vi "Create Legend.vi"(7 "Selection":i32, 9 "Colors[] (Use Default)":u32[](array[colorbox]), 10 "Font":T1, 11 "Labels[]":string[](array[string])) -> (2 "Legend Box Size":cluster{"Width":u32, "Height":u32}, 3 "Legend out":picture)   [LabVIEW 2018, in "PieChart.lvclass"]
uses:
  PieChart.lvclass
  <vilib>/picture/picture.llb/Draw True-Color Pixmap.vi
  <vilib>/Utility/miscctls.llb/LVFontTypeDef.ctl
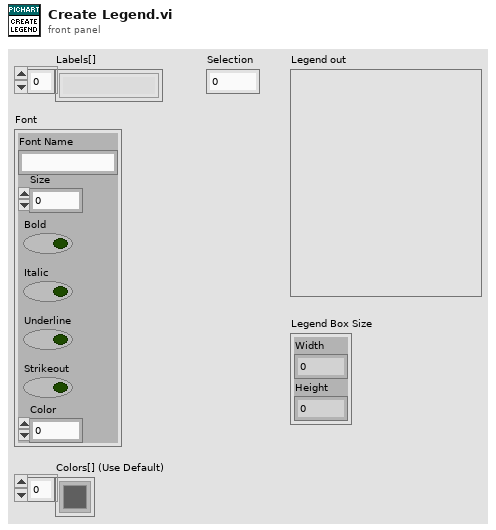
[diagram p1: front panel]
types:
  T1 = typedef "LVFontTypeDef.ctl" = cluster{"Font Name":string, "Size":u16, "Bold":bool, "Italic":bool, "Underline":bool, "Strikeout":bool, "Color":u32}
  T2 = cluster{"left":i16, "top":i16, "right":i16, "bottom":i16}
  T3 = enum16{"User-specified Font", "Application Font", "System Font", "Dialog Font"}
  T4 = cluster{"Font Name:":string, "Size":i16, "Strikeout?":bool, "Italic?":bool, "Underline?":bool, "Outline?":bool, "Shadow?":bool, "Bold?":bool}
  T5 = cluster{"left":u32, "top":u32, "right":u32, "bottom":u32}
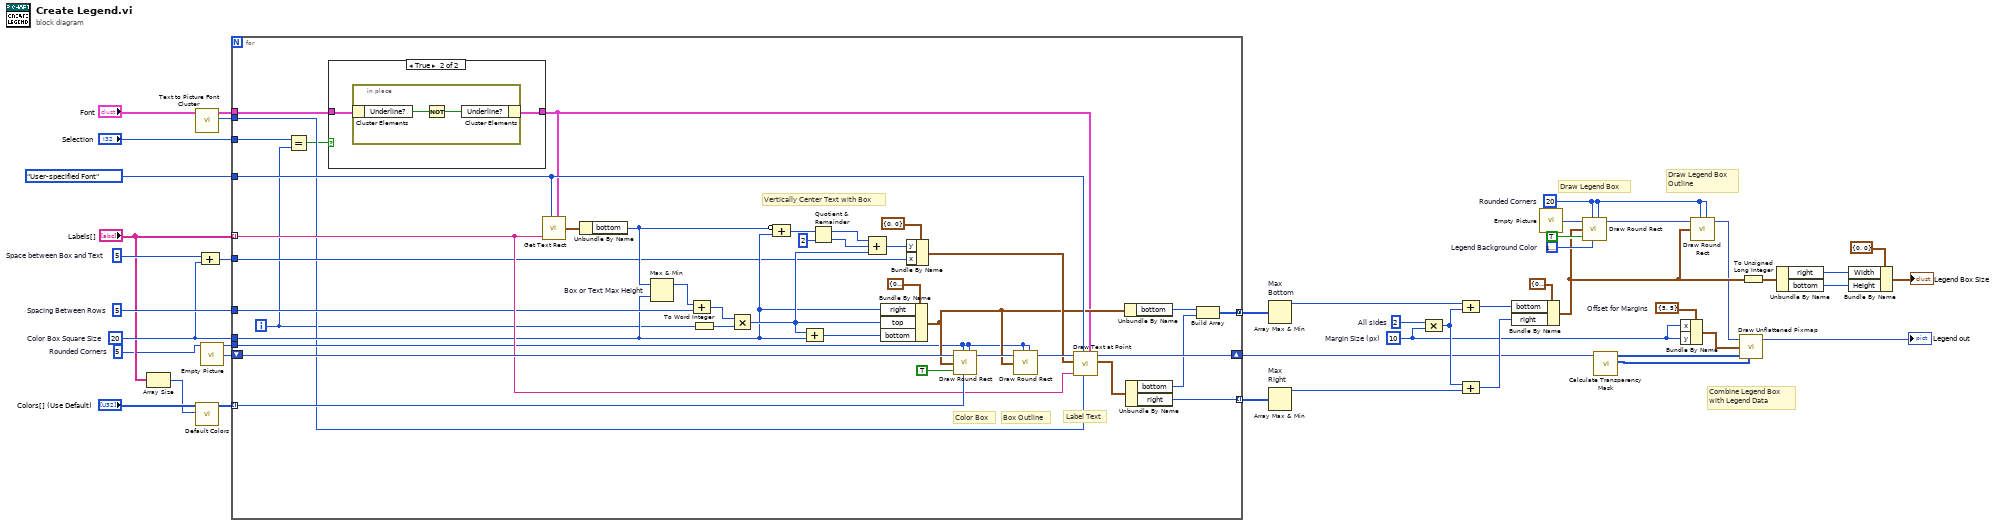
[diagram p0: block diagram]
diagram:
  w8 = i16 5  # Rounded Corners
  w9 = i16 20  # Rounded Corners
  w25 = i16 2  # All sides
  w30 = i16 5  # Space between Box and Text
  w31 = i16 20  # Color Box Square Size
  w32 = i16 5  # Spacing Between Rows
  w23 = cluster{"x":i16, "y":i16} {"x"=5, "y"=5}  # Offset for Margins
  w36 = u32 16777238  # Legend Background Color
  w21 = i16 10  # Margin Size (px)
  # "Draw Legend Box"
  # "Combine Legend Box\nwith Legend Data"
  # "Draw Legend Box\nOutline"
  n1 = Array Size(array="Labels[]") -> (size(s)=w10:i32)
  n2 = call "Text to Picture Font Cluster.vi"("Text Font Cluster"="Font") -> ("Color"=w5:u32, "Picture Font Cluster"=w6:T4)  [unwired: 9 in]
  n3 = call "Default Colors.vi"("Number of Entries"=w10, "Colors[] in"="Colors[] (Use Default)") -> ("Colors[] out"=w12:u32[])  [unwired: 9 in]
  n4 = call "Empty Picture"() -> ("empty picture"=w33:picture)
  n5 = Compound Arithmetic op=unknown(w30, w31) -> (w29:i16)
  n6 = for {
    tunnel: "Labels[]" -> [w71] mode=indexing
    tunnel: w12 -> [w82] mode=indexing
    shift-right: [w70] -> w4
    shift-left: w33 -> [w79]
    tunnel: T3."User-specified Font" ("desired font(Application)") -> [w74]
    tunnel: w6 -> [w46]
    tunnel: [w66] -> w41 mode=concatenating
    tunnel: [w52] -> w39 mode=indexing
    tunnel: w32 -> [w58]
    tunnel: w31 -> [w55]
    tunnel: w29 -> [w53]
    tunnel: w8 -> [w51]
    tunnel: w5 -> [w50]
    tunnel: "Selection" -> [w49]
    i -> [w47]
    # "Label Text"
    # "Box Outline"
    # "Color Box"
    # "Vertically Center Text with Box"
    n7 = Equal?(x=w49, y=w47) -> (x = y?=w45:bool)
    n8 = case shown="True" w45 {
      tunnel: w46 -> [w83 w85]
      tunnel: [w83 w84] -> w44
      frame False {
      }
      frame True {
        n9 = in-place {
          n10 = in-place-cluster #1(w85) -> ("Underline?"=w87:bool)
          n11 = Not(x=w87) -> (.not. x?=w86:bool)
          n12 = in-place-cluster #1("Underline?"=w86) -> (w84:T4)
        }
      }
    }
    n13 = call <vilib>:"Get Text Rect.vi"("desired font(Application)"=w74, "text"=w71, "[user-specified font]"=w44) -> ("rect"=w76:T2)  [unwired: 6 in]
    n14 = Unbundle By Name(w76) -> ("bottom"=w57:i16)
    n15 = Max & Min "Box or Text Max Height"(x=w57, y=w55) -> (max(x,y)=w56:i16)  [unwired: 1 out]
    n16 = To Word Integer(number=w47) -> (16bit integer=w59:i16)
    n17 = Compound Arithmetic op=ADD(w56, w58) -> (w48:i16)
    n18 = Multiply(x=w48, y=w59) -> (x*y=w60:i16)
    n19 = Compound Arithmetic op=ADD(invert w57, w55) -> (w64:i16)
    n20 = Compound Arithmetic op=ADD(w60, w55) -> (w78:i16)
    n21 = Quotient & Remainder(x=w64, y=i16 2) -> (x-y*floor(x/y)=w61:i16, floor(x/y)=w62:i16)
    n22 = Compound Arithmetic op=ADD(w61, w62, w60) -> (w65:i16)
    n23 = Bundle By Name(cluster=T2 {"left"=0, "top"=0, "right"=0, "bottom"=0} ("rect"), "right"=w55, "top"=w60, "bottom"=w78) -> (w68:T2)
    n24 = Bundle By Name(cluster=cluster{"x":i16, "y":i16} {"x"=0, "y"=0} ("origin"), "y"=w65, "x"=w53) -> (w72:cluster{"x":i16, "y":i16})
    n25 = call <vilib>:"Draw Round Rect.vi"("picture"=w79, "oval width"=w51, "rect"=w68, "fill?(F)"=TRUE, "color(black)"=w82, "oval height"=w51) -> ("new picture"=w77:picture)  [unwired: 3 in]
    n26 = call <vilib>:"Draw Round Rect.vi"("picture"=w77, "oval width"=w51, "rect"=w68, "oval height"=w51) -> ("new picture"=w75:picture)  [unwired: 5 in]
    n27 = call <vilib>:"Draw Text at Point.vi"("[user-specified font]"=w44, "text color(black)"=w50, "desired font(Application)"=w74, "text"=w71, "origin"=w72, "picture"=w75) -> ("text rect"=w69:T2, "new picture"=w70:picture)  [unwired: 4 in]
    n28 = Unbundle By Name(w68) -> ("bottom"=w54:i16)
    n29 = Unbundle By Name(w69) -> ("bottom"=w67:i16, "right"=w52:i16)
    n30 = Build Array(w54, w67) -> (w66:i16[])
  }
  n31 = Array Max & Min "Max\nBottom"(array=w41) -> (max value=w40:i16)  [unwired: 3 out]
  n32 = Array Max & Min "Max \nRight"(array=w39) -> (max value=w27:i16)  [unwired: 3 out]
  n33 = Compound Arithmetic op=MULTIPLY(w25, w21) -> (w24:i16)
  n34 = Compound Arithmetic op=ADD(w40, w24) -> (w38:i16)
  n35 = Compound Arithmetic op=ADD(w24, w27) -> (w26:i16)
  n36 = Bundle By Name(cluster=T2 {"left"=0, "top"=0, "right"=0, "bottom"=0} ("rect"), "bottom"=w38, "right"=w26) -> (w19:T2)
  n37 = call "Empty Picture"() -> ("empty picture"=w28:picture)
  n38 = call <vilib>:"Draw Round Rect.vi"("picture"=w28, "oval width"=w9, "rect"=w19, "fill?(F)"=TRUE, "color(black)"=w36, "oval height"=w9) -> ("new picture"=w35:picture)  [unwired: 3 in]
  n39 = call "Calculate Transparency Mask.vi"("Picture in"=w4) -> ("mask"=w2:u8[], "24-bit pixmap"=w3:u32[][])  [unwired: 8 in, 1 out]
  n40 = Bundle By Name(cluster=w23, "x"=w21, "y"=w21) -> (w22:cluster{"x":i16, "y":i16})
  n41 = call <vilib>:"Draw Round Rect.vi"("picture"=w35, "oval width"=w9, "rect"=w19, "oval height"=w9) -> ("new picture"=w14:picture)  [unwired: 5 in]
  n42 = call-poly <vilib>:"Draw Unflattened Pixmap.vi"("picture"=w14, "top left point(0, 0)"=w22, "data (RGB format)"=w3, "mask"=w2) -> ("new picture"=→"Legend out":picture)  [unwired: 5 in]
  n43 = To Unsigned Long Integer(number=w19) -> (unsigned 32bit integer=w15:T5)
  n44 = Unbundle By Name(w15) -> ("right"=w18:u32, "bottom"=w16:u32)
  n45 = Bundle By Name(cluster=cluster{"Width":u32, "Height":u32} {"Width"=0, "Height"=0} ("Legend Box Size"), "Width"=w18, "Height"=w16) -> (→"Legend Box Size":cluster{"Width":u32, "Height":u32})
